vi "Config-Chan-VSUs-Sweep.vi"(0 "VISA session":refnum<visa-resource-name>, 1 "VSU1 function":i32(slide) max=4 scale=0.0..4.0, 2 "VSU2 V name \n(max 6 chars)":string, 5 "VSU1 standby":bool, 9 "VSU2 standby":bool, 11 "error in (no error)":errorcluster, 12 "VSU2 function":i32(slide) max=4 scale=0.0..4.0, 13 "VSU1 V name \n(max 6 chars)":string) -> (4 "VISA resource name out":refnum<visa-resource-name>, 15 "error out":errorcluster)   [LabVIEW 2016, in "Agilent 415X Series.lvlib"]
doc: "This VI configures both VSUs in sample measurement mode. \n\nThis VI corresponds to the Channel Definition Page (when Measurement Mode is set to SAMPLING) of the instrument. In general, it allows every setting change that can be made via the instrument's front panel although the change may cause a setting conflict when a measurement is initialied."
uses:
  Agilent 415X Series.lvlib
panel:
  # "* This VI does NOT report all setting errors. Error \nchecking must be done when a measurement is initialized."
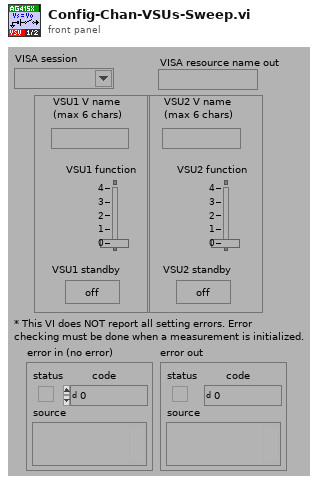
[diagram p1: front panel]
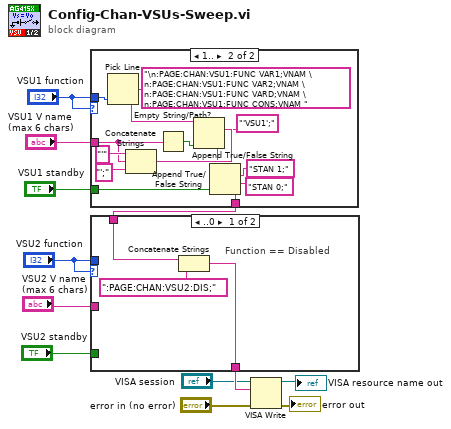
[diagram p0: block diagram]
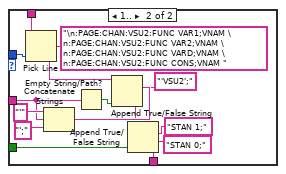
[diagram p2: hidden frame]
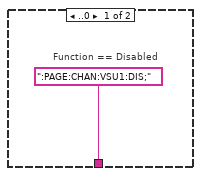
[diagram p3: hidden frame]
diagram:
  n1 = case shown="1.." "VSU1 function" {
    tunnel: "VSU1 V name \n(max 6 chars)" -> [_ w25]
    tunnel: "VSU1 standby" -> [_ w20]
    tunnel: [":PAGE:CHAN:VSU1:DIS;" w21] -> w5
    tunnel: "VSU1 function" -> [_ w18]
    frame ..0 {
      # "Function == Disabled"
    }
    frame 1.. {
      n2 = Pick Line(multi-line string="\n:PAGE:CHAN:VSU1:FUNC VAR1;VNAM \n:PAGE:CHAN:VSU1:FUNC VAR2;VNAM \n:PAGE:CHAN:VSU1:FUNC VARD;VNAM \n:PAGE:CHAN:VSU1:FUNC CONS;VNAM ", line index=w18) -> (output string=w14:string)  [unwired: 1 in]
      n3 = Concatenate Strings("'", w25, "';") -> (w24:string)
      n4 = Empty String/Path?(string/path=w25) -> (empty?=w27:bool)
      n5 = Append True/False String(1:w27, 2:w24, 3:"'VSU1';", 4:w14) -> (0:w16:string)
      n6 = Append True/False String(1:w20, 2:"STAN 0;", 3:"STAN 1;", 4:w16) -> (0:w21:string)
    }
  }
  n7 = case shown="..0" "VSU2 function" {
    tunnel: "VSU2 V name \n(max 6 chars)" -> [_ w43]
    tunnel: "VSU2 standby" -> [_ w38]
    tunnel: [w30 w39] -> w4
    tunnel: "VSU2 function" -> [_ w36]
    tunnel: w5 -> [w28 w33]
    frame ..0 {
      # "Function == Disabled"
      n8 = Concatenate Strings(w28, ":PAGE:CHAN:VSU2:DIS;") -> (w30:string)
    }
    frame 1.. {
      n9 = Pick Line(string ("")=w33, multi-line string="\n:PAGE:CHAN:VSU2:FUNC VAR1;VNAM \n:PAGE:CHAN:VSU2:FUNC VAR2;VNAM \n:PAGE:CHAN:VSU2:FUNC VARD;VNAM \n:PAGE:CHAN:VSU2:FUNC CONS;VNAM ", line index=w36) -> (output string=w31:string)
      n10 = Concatenate Strings("'", w43, "';") -> (w42:string)
      n11 = Empty String/Path?(string/path=w43) -> (empty?=w45:bool)
      n12 = Append True/False String(1:w45, 2:w42, 3:"'VSU2';", 4:w31) -> (0:w34:string)
      n13 = Append True/False String(1:w38, 2:"STAN 0;", 3:"STAN 1;", 4:w34) -> (0:w39:string)
    }
  }
  n14 = VISA Write(VISA resource name="VISA session", write buffer=w4, error in (no error)="error in (no error)") -> (VISA resource name out=→"VISA resource name out":refnum<visa-resource-name>, error out=→"error out":errorcluster)  [unwired: 1 out]
